vi "Autonomous Independent.vi"   [LabVIEW 2017]
doc: "This VI is called when autonomous begins, and will automatically be terminated when autonomous ends. You can carry out timed or sensor driven robot movement independently without needing to return to the caller."
uses:
  <vilib>/Rock Robotics/WPI/Utilities/WPI_GetSetVariantRefNum.vi
  <vilib>/Rock Robotics/Network Tables/NT Write Numeric Array.vi
  <vilib>/Rock Robotics/Network Tables/NT Read String.vi
  <vilib>/Rock Robotics/WPI/RobotDrive/WPI_RobotDriveMecanumDrive_Cartesian.vi
types:
  T1 = typedef "WPI_JoystickDevRef.ctl" = cluster{"Device":T2}
  T2 = typedef "WPI_JoystickDeviceEnum.ctl" = enum16{"USB 0", "USB 1", "USB 2", "USB 3", "USB 4", "USB 5"}
  T3 = typedef "WPI_RobotDriveDevRef.ctl" = cluster{"DevStatus":errorcluster, "Motors[]":T4[], "Square Inputs":bool, "Max Output":dbl}
  T4 = typedef "WPI_MotorControlDeviceRef.ctl" = cluster{"DeviceStatus":errorcluster, "Type":T5, "PWM":cluster{"PWM Channel":T6, "DeadBand":T7}, "CAN":cluster{"Device Number":u8, "SetOutput VI Ref":variant, "GetOutput VI Ref":variant, "Enable VI Ref":variant, "Disable VI Ref":variant, "Data":variant}, "Invert":bool, "DIO PWM":cluster{"PWM \"Enable\" Channel":T6, "DIOChannel":T8, "PWM Rate":dbl}}
  T5 = typedef "WPI_MotorControlType.ctl" = enum16{"PWM", "CAN", "DIO PWM"}
  T6 = typedef "FPGA_DIOPWMChannel.ctl" = enum8{"PWM 0", "PWM 1", "PWM 2", "PWM 3", "PWM 4", "PWM 5", "PWM 6", "PWM 7", "PWM 8", "PWM 9", "PWM MXP 0", "PWM MXP 1", "PWM MXP 2", "PWM MXP 3", "PWM MXP 4", "PWM MXP 5", "PWM MXP 6", "PWM MXP 7", "PWM MXP 8", "PWM MXP 9", "Invalid"}
  T7 = typedef "WPI_PWMDeadband.ctl" = cluster{"Name":string, "maxPositivePwm":i32, "minPositivePwm":i32, "centerPwm":i32, "maxNegativePwm":i32, "minNegativePwm":i32, "angularRange":u16}
  T8 = typedef "FPGA_DIOChannel.ctl" = enum8{"DIO 0", "DIO 1", "DIO 2", "DIO 3", "DIO 4", "DIO 5", "DIO 6", "DIO 7", "DIO 8", "DIO 9", "DIO MXP 0", "DIO MXP 1", "DIO MXP 2", "DIO MXP 3", "DIO MXP 4", "DIO MXP 5", "DIO MXP 6", "DIO MXP 7", "DIO MXP 8", "DIO MXP 9", "DIO MXP 10", "DIO MXP 11", "DIO MXP 12", "DIO MXP 13", "DIO MXP 14", "DIO MXP 15", "SPI Port CS1", "SPI Port CS2", "SPI Port CS3", "SPI Port MISO", "SPI Port MOSI", "Invalid"}
  T9 = typedef "WPI_EncoderDevRef.ctl" = cluster{"DevStatus":errorcluster, "EncoderIndex":T10, "CounterIndex":T11, "DistancePerCount":dbl, "Decoding Type":T12}
  T10 = typedef "FPGA_EncoderIdx.ctl" = enum8{"Enc 0", "Enc 1", "Enc 2", "Enc 3", "Enc 4", "Enc 5", "Enc 6", "Enc 7", "Invalid"}
  T11 = typedef "FPGA_CounterCtrSystemIndex.ctl" = enum8{"Ctr 0", "Ctr 1", "Ctr 2", "Ctr 3", "Ctr 4", "Ctr 5", "Ctr 6", "Ctr 7", "Invalid"}
  T12 = typedef "WPI_EncoderType.ctl" = enum16{"1x", "2x", "4x"}
  T13 = typedef "WPI_GyroDevRef.ctl" = cluster{"DevStatus":errorcluster, "Analog Channel":T14, "Gain (VoltsPerDegree/Second)":dbl, "Gyro Type":enum16{"Analog", "XRS450"}, "Handle":i32, "SPI Bus":T15, "Device Found":bool, "Sample Rate":dbl, "Calibrate On Open":bool, "Offset":dbl}
  T14 = typedef "FPGA_AIChannel.ctl" = enum8{"AI 0", "AI 1", "AI 2", "AI 3", "AI MXP 0", "AI MXP 1", "AI MXP 2", "AI MXP 3", "Invalid"}
  T15 = typedef "spi_bus.ctl" = enum16{"SPI On-Board, CS0", "SPI On-Board, CS1", "SPI On-Board, CS2", "SPI On-Board, CS3", "SPI MXP", "Invalid"}
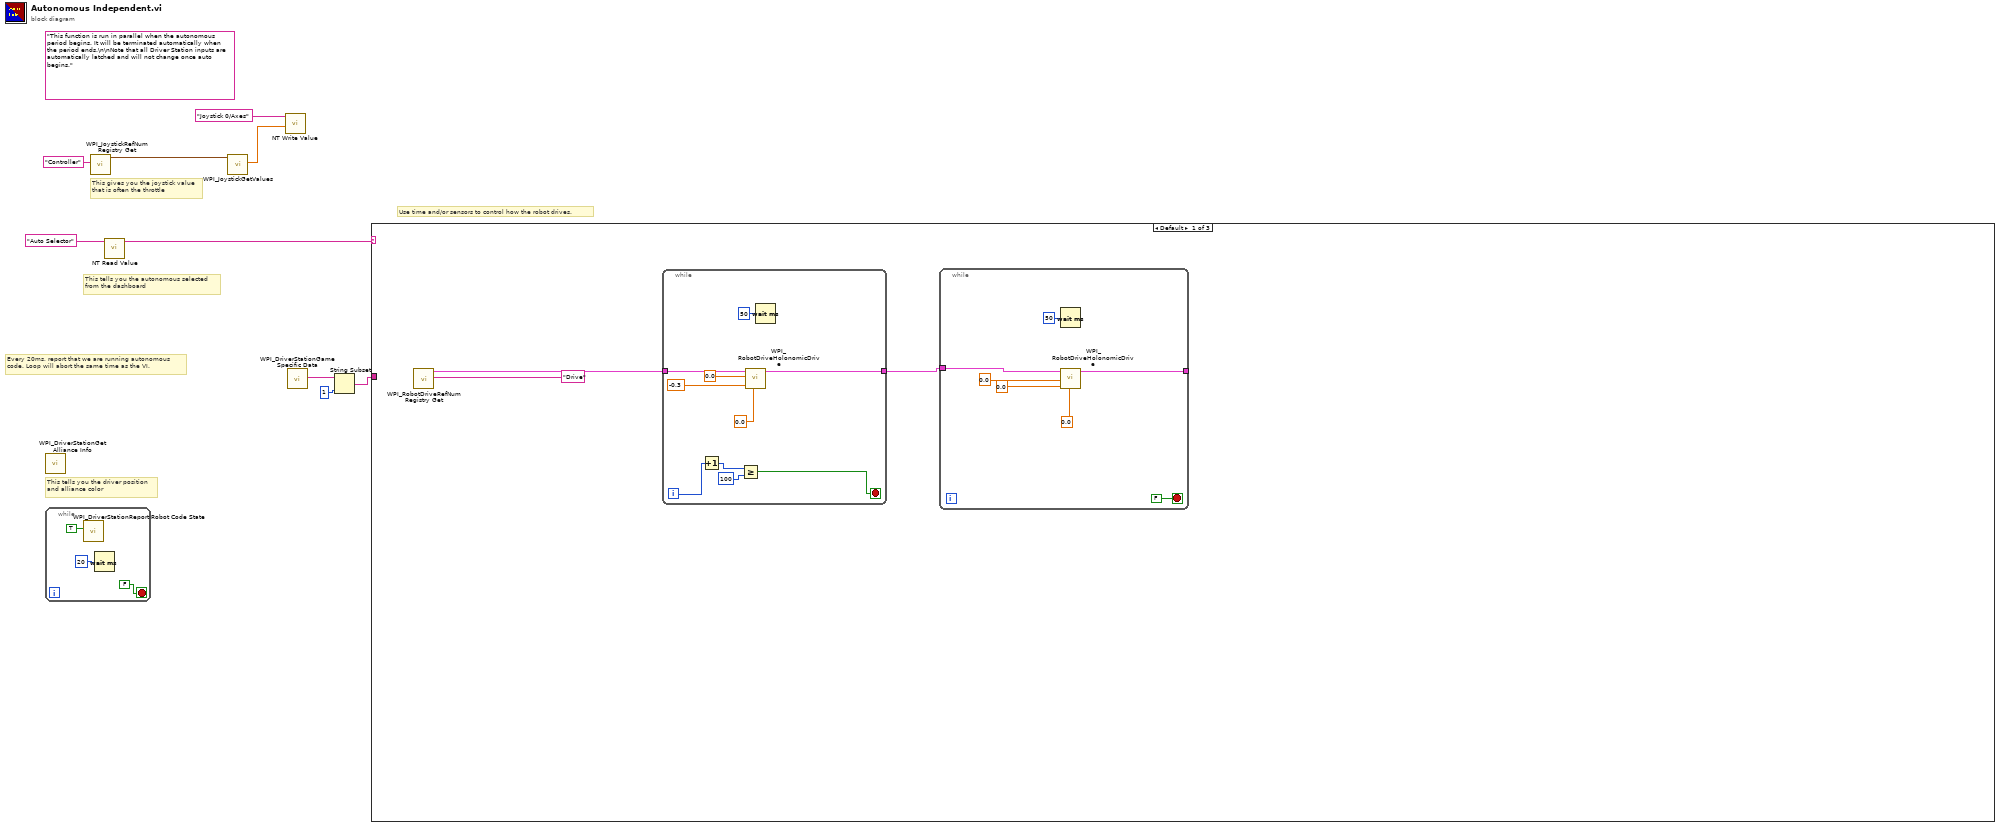
[diagram p0: block diagram]
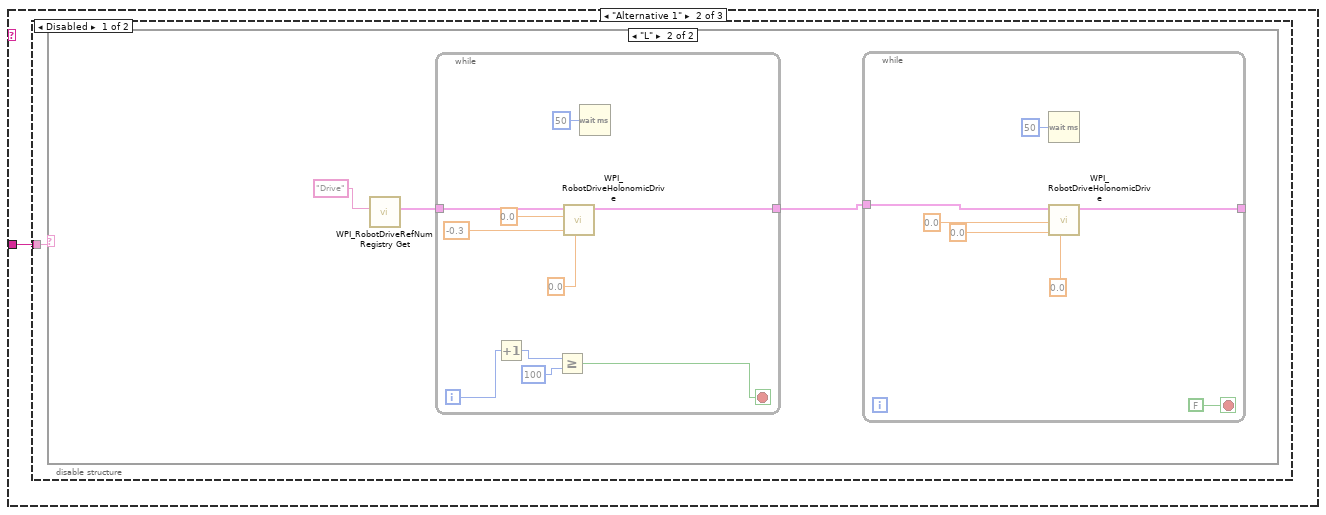
[diagram p2: hidden frame]
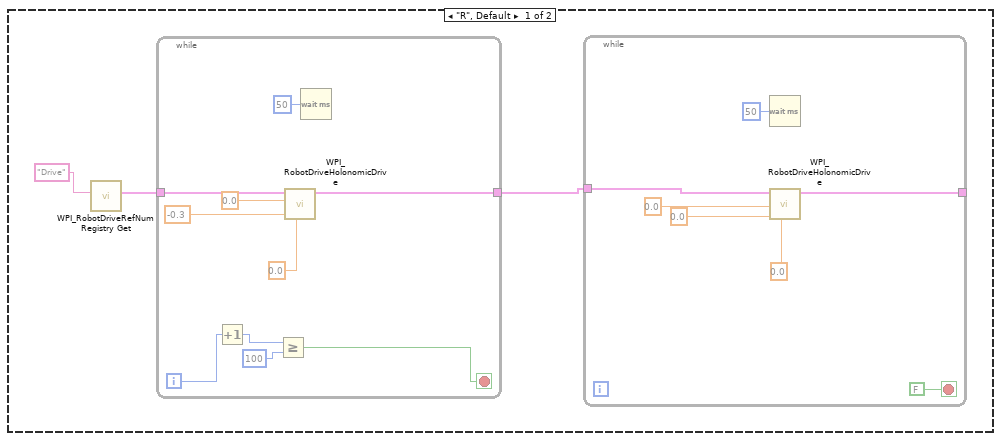
[diagram p3: hidden frame]
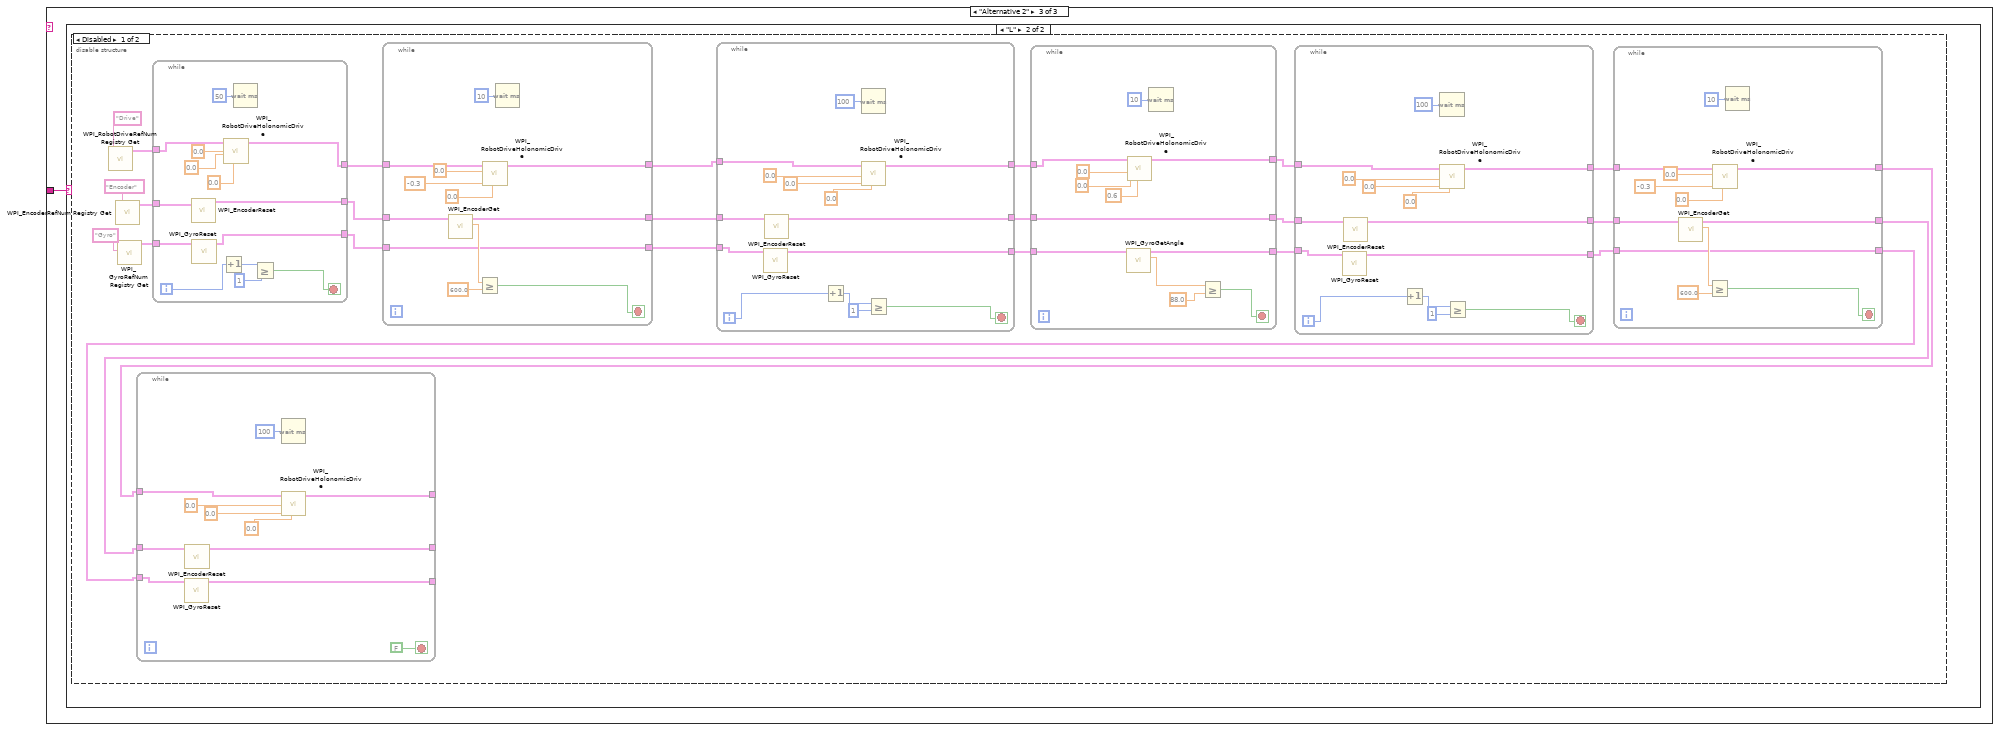
[diagram p5: hidden frame]
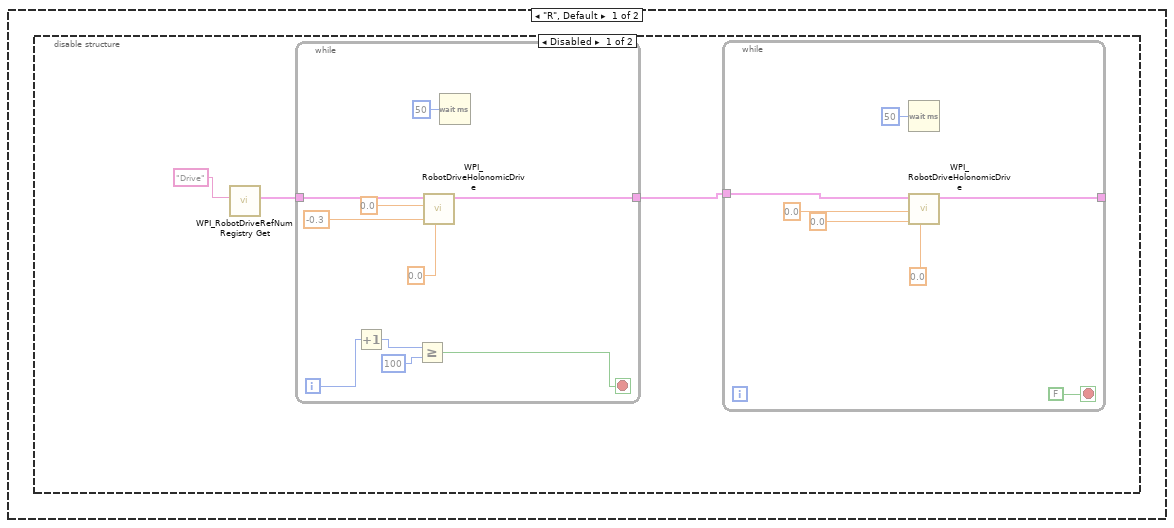
[diagram p6: hidden frame]
diagram:
  (unwired) "This function is run in parallel when the autonomous period begins. It will be terminated automatically when the period ends.\n\nNote that all Driver Station inputs are automatically latched and will not change once auto begins."
  # "This tells you the autonomous selected\nfrom the dashboard"
  # "Use time and/or sensors to control how the robot drives."
  # "Every 20ms, report that we are running autonomous\ncode. Loop will abort the same time as the VI."
  # "This gives you the joystick value\nthat is often the throttle"
  # "This tells you the driver position\nand alliance color"
  n1 = call <vilib>:"WPI_DriverStationGet Alliance Info.vi"() -> ()  [unwired: 12 out]
  n2 = while {
    stop <- FALSE stop-if-true
    n3 = call <vilib>:"WPI_DriverStationReport Robot Code State.vi"("Autonomous"=TRUE) -> ()  [unwired: 10 in, 1 out]
    n4 = Wait (ms)(milliseconds to wait=u32 20) -> ()  [unwired: 1 out]
  }
  n5 = call <vilib>:"WPI_JoystickRefNum Registry Get.vi"("refnum name"="Controller") -> ("JoystickDevRef"=w8:T1)  [unwired: 1 in, 9 out]
  n6 = call-poly <vilib>:"NT Read Value.vi"("Name"="Auto Selector") -> ("String"=w4:string)  [unwired: 9 in, 1 out]
  n7 = call <vilib>:"WPI_JoystickGetValues.vi"("JoystickDevRef"=w8) -> ("Axes"=w7:dbl[])  [unwired: 6 in, 4 out]
  n8 = call-poly <vilib>:"NT Write Value.vi"("Numeric Array"=w7, "Name"="Joystick 0/Axes") -> ()  [unwired: 9 in, 1 out]
  n9 = call <vilib>:"WPI_DriverStationGame Specific Data.vi"() -> ("Game Specific Data"=w2:string)  [unwired: 11 in]
  n10 = String Subset(string=w2, length (rest)=1 ("length (rest)")) -> (substring=w1:string)  [unwired: 1 in]
  n11 = case shown="Default" w4 {
    tunnel: w1 -> [_ w33 w75]
    frame Default {
      n12 = call <vilib>:"WPI_RobotDriveRefNum Registry Get.vi"("refnum name"="Drive") -> ("RobotDriveDevRef"=w14:T3)  [unwired: 9 in, 1 out]
      n13 = while {
        tunnel: w14 -> [w32]
        tunnel: [w23] -> w15
        i -> [w27]
        stop <- w24 stop-if-true
        n14 = Increment(x=w27) -> (x+1=w26:i32)
        n15 = Greater Or Equal?(x=w26, y=100) -> (x >= y?=w24:bool)
        n16 = call-poly <vilib>:"WPI_RobotDriveHolonomicDrive.vi"("Rotation"=0.0, "Y"=-0.3, "X"=0.0, "RobotDriveDevRef"=w32) -> ("RobotDriveDevRef"=w23:T3)  [unwired: 5 in, 2 out]
        n17 = Wait (ms)(milliseconds to wait=u32 50) -> ()  [unwired: 1 out]
      }
      n18 = while {
        tunnel: w15 -> [w22]
        tunnel: [w21] -> _
        stop <- FALSE stop-if-true
        n19 = Wait (ms)(milliseconds to wait=u32 50) -> ()  [unwired: 1 out]
        n20 = call-poly <vilib>:"WPI_RobotDriveHolonomicDrive.vi"("Rotation"=0.0, "Y"=0.0, "X"=0.0, "RobotDriveDevRef"=w22) -> ("RobotDriveDevRef"=w21:T3)  [unwired: 5 in, 2 out]
      }
    }
    frame "Alternative 1" {
      n21 = disable-structure shown="Disabled" {
        disable-tunnel: w33 -> [w34 _]
        frame Disabled {
          n22 = case shown="\"L\"" w34 {
            frame "R", Default {
              n23 = call <vilib>:"WPI_RobotDriveRefNum Registry Get.vi"("refnum name"="Drive") -> ("RobotDriveDevRef"=w37:T3)  [unwired: 9 in, 1 out]
              n24 = while {
                tunnel: w37 -> [w54]
                tunnel: [w45] -> w36
                i -> [w49]
                stop <- w46 stop-if-true
                n25 = Increment(x=w49) -> (x+1=w48:i32)
                n26 = Greater Or Equal?(x=w48, y=100) -> (x >= y?=w46:bool)
                n27 = call-poly <vilib>:"WPI_RobotDriveHolonomicDrive.vi"("Rotation"=0.0, "Y"=-0.3, "X"=0.0, "RobotDriveDevRef"=w54) -> ("RobotDriveDevRef"=w45:T3)  [unwired: 5 in, 2 out]
                n28 = Wait (ms)(milliseconds to wait=u32 50) -> ()  [unwired: 1 out]
              }
              n29 = while {
                tunnel: w36 -> [w44]
                tunnel: [w43] -> _
                stop <- FALSE stop-if-true
                n30 = Wait (ms)(milliseconds to wait=u32 50) -> ()  [unwired: 1 out]
                n31 = call-poly <vilib>:"WPI_RobotDriveHolonomicDrive.vi"("Rotation"=0.0, "Y"=0.0, "X"=0.0, "RobotDriveDevRef"=w44) -> ("RobotDriveDevRef"=w43:T3)  [unwired: 5 in, 2 out]
              }
            }
            frame "L" {
              n32 = call <vilib>:"WPI_RobotDriveRefNum Registry Get.vi"("refnum name"="Drive") -> ("RobotDriveDevRef"=w57:T3)  [unwired: 9 in, 1 out]
              n33 = while {
                tunnel: w57 -> [w74]
                tunnel: [w65] -> w56
                i -> [w69]
                stop <- w66 stop-if-true
                n34 = Increment(x=w69) -> (x+1=w68:i32)
                n35 = Greater Or Equal?(x=w68, y=100) -> (x >= y?=w66:bool)
                n36 = call-poly <vilib>:"WPI_RobotDriveHolonomicDrive.vi"("Rotation"=0.0, "Y"=-0.3, "X"=0.0, "RobotDriveDevRef"=w74) -> ("RobotDriveDevRef"=w65:T3)  [unwired: 5 in, 2 out]
                n37 = Wait (ms)(milliseconds to wait=u32 50) -> ()  [unwired: 1 out]
              }
              n38 = while {
                tunnel: w56 -> [w64]
                tunnel: [w63] -> _
                stop <- FALSE stop-if-true
                n39 = Wait (ms)(milliseconds to wait=u32 50) -> ()  [unwired: 1 out]
                n40 = call-poly <vilib>:"WPI_RobotDriveHolonomicDrive.vi"("Rotation"=0.0, "Y"=0.0, "X"=0.0, "RobotDriveDevRef"=w64) -> ("RobotDriveDevRef"=w63:T3)  [unwired: 5 in, 2 out]
              }
            }
          }
        }
        frame Enabled {
        }
      }
    }
    frame "Alternative 2" {
      n41 = case shown="\"L\"" w75 {
        frame "R", Default {
          n42 = disable-structure shown="Disabled" {
            frame Disabled {
              n43 = call <vilib>:"WPI_RobotDriveRefNum Registry Get.vi"("refnum name"="Drive") -> ("RobotDriveDevRef"=w78:T3)  [unwired: 9 in, 1 out]
              n44 = while {
                tunnel: w78 -> [w95]
                tunnel: [w86] -> w77
                i -> [w90]
                stop <- w87 stop-if-true
                n45 = Increment(x=w90) -> (x+1=w89:i32)
                n46 = Greater Or Equal?(x=w89, y=100) -> (x >= y?=w87:bool)
                n47 = call-poly <vilib>:"WPI_RobotDriveHolonomicDrive.vi"("Rotation"=0.0, "Y"=-0.3, "X"=0.0, "RobotDriveDevRef"=w95) -> ("RobotDriveDevRef"=w86:T3)  [unwired: 5 in, 2 out]
                n48 = Wait (ms)(milliseconds to wait=u32 50) -> ()  [unwired: 1 out]
              }
              n49 = while {
                tunnel: w77 -> [w85]
                tunnel: [w84] -> _
                stop <- FALSE stop-if-true
                n50 = Wait (ms)(milliseconds to wait=u32 50) -> ()  [unwired: 1 out]
                n51 = call-poly <vilib>:"WPI_RobotDriveHolonomicDrive.vi"("Rotation"=0.0, "Y"=0.0, "X"=0.0, "RobotDriveDevRef"=w85) -> ("RobotDriveDevRef"=w84:T3)  [unwired: 5 in, 2 out]
              }
            }
            frame Enabled {
            }
          }
        }
        frame "L" {
          n52 = disable-structure shown="Disabled" {
            frame Disabled {
              n53 = call <vilib>:"WPI_RobotDriveRefNum Registry Get.vi"("refnum name"="Drive") -> ("RobotDriveDevRef"=w116:T3)  [unwired: 9 in, 1 out]
              n54 = call <vilib>:"WPI_EncoderRefNum Registry Get.vi"("refnum name"="Encoder") -> ("EncoderDevRef"=w113:T9)  [unwired: 9 in, 1 out]
              n55 = call <vilib>:"WPI_GyroRefNum Registry Get.vi"("refnum name"="Gyro") -> ("GyroDevRef"=w112:T13)  [unwired: 9 in, 1 out]
              n56 = while {
                tunnel: [w181] -> w118
                tunnel: w116 -> [w182]
                tunnel: w113 -> [w178]
                tunnel: w112 -> [w177]
                tunnel: [w176] -> w111
                tunnel: [w175] -> w110
                i -> [w172]
                stop <- w169 stop-if-true
                n57 = call <vilib>:"WPI_EncoderReset.vi"("EncoderDevRef"=w178) -> ("EncoderDevRef"=w176:T9)  [unwired: 9 in, 1 out]
                n58 = call <vilib>:"WPI_GyroReset.vi"("GyroDevRef"=w177) -> ("GyroDevRef"=w175:T13)  [unwired: 9 in, 1 out]
                n59 = Increment(x=w172) -> (x+1=w171:i32)
                n60 = call-poly <vilib>:"WPI_RobotDriveHolonomicDrive.vi"("Rotation"=0.0, "Y"=0.0, "X"=0.0, "RobotDriveDevRef"=w182) -> ("RobotDriveDevRef"=w181:T3)  [unwired: 5 in, 2 out]
                n61 = Wait (ms)(milliseconds to wait=u32 50) -> ()  [unwired: 1 out]
                n62 = Greater Or Equal?(x=w171, y=1) -> (x >= y?=w169:bool)
              }
              n63 = while {
                tunnel: w118 -> [w208]
                tunnel: [w202] -> w119
                tunnel: w111 -> [w201]
                tunnel: w110 -> [w198]
                tunnel: [w198] -> w108
                tunnel: [w197] -> w109
                stop <- w203 stop-if-true
                n64 = call <vilib>:"WPI_EncoderGet.vi"("EncoderDevRef"=w201) -> ("Distance"=w200:dbl, "EncoderDevRef"=w197:T9)  [unwired: 5 in, 4 out]
                n65 = Greater Or Equal?(x=w200, y=600.0) -> (x >= y?=w203:bool)
                n66 = call-poly <vilib>:"WPI_RobotDriveHolonomicDrive.vi"("Rotation"=0.0, "Y"=-0.3, "X"=0.0, "RobotDriveDevRef"=w208) -> ("RobotDriveDevRef"=w202:T3)  [unwired: 5 in, 2 out]
                n67 = Wait (ms)(milliseconds to wait=u32 10) -> ()  [unwired: 1 out]
              }
              n68 = while {
                tunnel: w119 -> [w196]
                tunnel: [w195] -> w107
                tunnel: w109 -> [w186]
                tunnel: w108 -> [w185]
                tunnel: [w184] -> w106
                tunnel: [w183] -> w105
                i -> [w190]
                stop <- w187 stop-if-true
                n69 = call <vilib>:"WPI_GyroReset.vi"("GyroDevRef"=w185) -> ("GyroDevRef"=w183:T13)  [unwired: 9 in, 1 out]
                n70 = call <vilib>:"WPI_EncoderReset.vi"("EncoderDevRef"=w186) -> ("EncoderDevRef"=w184:T9)  [unwired: 9 in, 1 out]
                n71 = Increment(x=w190) -> (x+1=w189:i32)
                n72 = Wait (ms)(milliseconds to wait=u32 100) -> ()  [unwired: 1 out]
                n73 = call-poly <vilib>:"WPI_RobotDriveHolonomicDrive.vi"("Rotation"=0.0, "Y"=0.0, "X"=0.0, "RobotDriveDevRef"=w196) -> ("RobotDriveDevRef"=w195:T3)  [unwired: 5 in, 2 out]
                n74 = Greater Or Equal?(x=w189, y=1) -> (x >= y?=w187:bool)
              }
              n75 = while {
                tunnel: w107 -> [w167]
                tunnel: w106 -> [w165]
                tunnel: w105 -> [w164]
                tunnel: [w166] -> w104
                tunnel: [w165] -> w103
                tunnel: [w163] -> w102
                stop <- w160 stop-if-true
                n76 = call <vilib>:"WPI_GyroGetAngle.vi"("GyroDevRef"=w164) -> ("Angle"=w162:dbl, "GyroDevRef"=w163:T13)  [unwired: 6 in, 3 out]
                n77 = call-poly <vilib>:"WPI_RobotDriveHolonomicDrive.vi"("Rotation"=0.6, "Y"=0.0, "X"=0.0, "RobotDriveDevRef"=w167) -> ("RobotDriveDevRef"=w166:T3)  [unwired: 5 in, 2 out]
                n78 = Wait (ms)(milliseconds to wait=u32 10) -> ()  [unwired: 1 out]
                n79 = Greater Or Equal?(x=w162, y=88.0) -> (x >= y?=w160:bool)
              }
              n80 = while {
                tunnel: w104 -> [w156]
                tunnel: [w155] -> w101
                tunnel: w103 -> [w146]
                tunnel: w102 -> [w145]
                tunnel: [w144] -> w100
                tunnel: [w143] -> w99
                i -> [w150]
                stop <- w147 stop-if-true
                n81 = call <vilib>:"WPI_GyroReset.vi"("GyroDevRef"=w145) -> ("GyroDevRef"=w143:T13)  [unwired: 9 in, 1 out]
                n82 = call <vilib>:"WPI_EncoderReset.vi"("EncoderDevRef"=w146) -> ("EncoderDevRef"=w144:T9)  [unwired: 9 in, 1 out]
                n83 = Increment(x=w150) -> (x+1=w149:i32)
                n84 = Wait (ms)(milliseconds to wait=u32 100) -> ()  [unwired: 1 out]
                n85 = call-poly <vilib>:"WPI_RobotDriveHolonomicDrive.vi"("Rotation"=0.0, "Y"=0.0, "X"=0.0, "RobotDriveDevRef"=w156) -> ("RobotDriveDevRef"=w155:T3)  [unwired: 5 in, 2 out]
                n86 = Greater Or Equal?(x=w149, y=1) -> (x >= y?=w147:bool)
              }
              n87 = while {
                tunnel: w101 -> [w142]
                tunnel: [w136] -> w98
                tunnel: w100 -> [w135]
                tunnel: w99 -> [w132]
                tunnel: [w132] -> w96
                tunnel: [w131] -> w97
                stop <- w137 stop-if-true
                n88 = call <vilib>:"WPI_EncoderGet.vi"("EncoderDevRef"=w135) -> ("Distance"=w134:dbl, "EncoderDevRef"=w131:T9)  [unwired: 5 in, 4 out]
                n89 = Greater Or Equal?(x=w134, y=600.0) -> (x >= y?=w137:bool)
                n90 = call-poly <vilib>:"WPI_RobotDriveHolonomicDrive.vi"("Rotation"=0.0, "Y"=-0.3, "X"=0.0, "RobotDriveDevRef"=w142) -> ("RobotDriveDevRef"=w136:T3)  [unwired: 5 in, 2 out]
                n91 = Wait (ms)(milliseconds to wait=u32 10) -> ()  [unwired: 1 out]
              }
              n92 = while {
                tunnel: w98 -> [w130]
                tunnel: [w129] -> _
                tunnel: w97 -> [w124]
                tunnel: w96 -> [w123]
                tunnel: [w122] -> _
                tunnel: [w121] -> _
                stop <- FALSE stop-if-true
                n93 = call <vilib>:"WPI_GyroReset.vi"("GyroDevRef"=w123) -> ("GyroDevRef"=w121:T13)  [unwired: 9 in, 1 out]
                n94 = call <vilib>:"WPI_EncoderReset.vi"("EncoderDevRef"=w124) -> ("EncoderDevRef"=w122:T9)  [unwired: 9 in, 1 out]
                n95 = Wait (ms)(milliseconds to wait=u32 100) -> ()  [unwired: 1 out]
                n96 = call-poly <vilib>:"WPI_RobotDriveHolonomicDrive.vi"("Rotation"=0.0, "Y"=0.0, "X"=0.0, "RobotDriveDevRef"=w130) -> ("RobotDriveDevRef"=w129:T3)  [unwired: 5 in, 2 out]
              }
            }
            frame Enabled {
            }
          }
        }
      }
    }
  }
